vi "set_scanners.vi"(8 "error in (no error)":errorcluster, 10 "scanners":refnum<class "GenericSignalWriter.lvclass">[](array[class]), 11 "ScanHeadAK130114ResonanceFlexRIO in":refnum<class "ScanHeadAK130114ResonanceFlexRIO.lvclass">) -> (0 "error out":errorcluster, 3 "ScanHeadAK130114ResonanceFlexRIO out":refnum<class "ScanHeadAK130114ResonanceFlexRIO.lvclass">)   [LabVIEW 2010, in "ScanHeadAK130114ResonanceFlexRIO.lvclass"]
uses:
  ScanHeadAK130114ResonanceFlexRIO.lvclass
  SignalWriter/GenericSignalWriter/GenericSignalWriter/GenericSignalWriter.lvclass
  ScanHeadAK130114ResonanceFlexRIO.lvclass/ScanHeadAK130114ResonanceFlexRIO.ctl
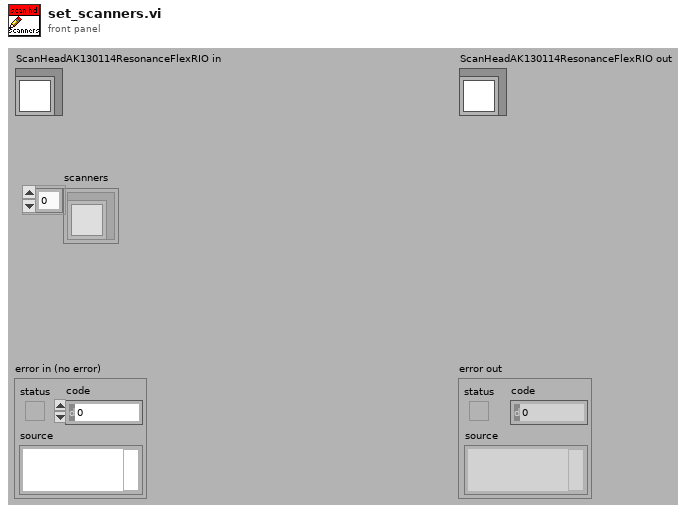
[diagram p1: front panel]
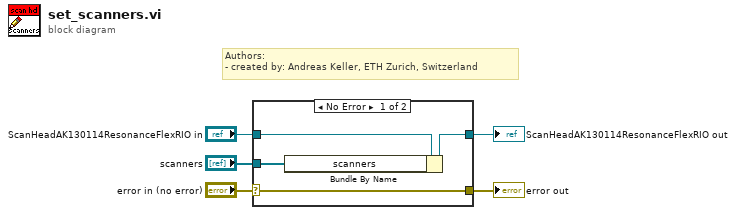
[diagram p0: block diagram]
diagram:
  # "Authors: \n- created by: Andreas Keller, ETH Zurich, Switzerland"
  n1 = case shown="No Error" "error in (no error)" {
    selector: "error in (no error)" -> [w9 w11]
    tunnel: [w9 w11] -> w4
    tunnel: [w7 w10] -> w2
    tunnel: "ScanHeadAK130114ResonanceFlexRIO in" -> [w8 w10]
    tunnel: "scanners" -> [w6 _]
    frame No Error {
      n2 = Bundle By Name(cluster=w8, "scanners"=w6) -> (w7:refnum<class "ScanHeadAK130114ResonanceFlexRIO.lvclass">)
    }
    frame Error {
    }
  }
  "error out" <- w4
  "ScanHeadAK130114ResonanceFlexRIO out" <- w2
